vi "DataViewer_Transport.vi"() -> ()   [LabVIEW 2019]
uses:
  <userlib>/LevyLab/XY Utilities/subVIs/Waveform to XY (multiple).vi
  <userlib>/LevyLab/XY Utilities/subVIs/Waveform to XY (single).vi
  <vilib>/Waveform/WDTOps.llb/Waveform to XY Pairs.vi
  <vilib>/Waveform/WDTOps.llb/WDT Waveform to XY Pairs DBL.vi
  <userlib>/LevyLab/XY Utilities/xy_utilities.lvlib
panel:
  in  "Excitation (V)":dbl format="%#_6p"
  in  "Plot XG":bool
  in  "Plot XR":bool
  in  "V-":u16(ring) items=["", "Time", "Temperature", "AO1", "AO2", "AO3", "AO4", "AO5", "AO6", "AO7", "AO8", "AO9", "AO10", "AI1", "AI2", "AI3", "AI4", "AI5", "AI6", "AI7", "AI8", "AI9", "AI10", "X1", "X2", "X3", "X4", "X5", "X6", "X7", "X8", "X9", "X10", "Y1", "Y2", "Y3", "Y4", "Y5", "Y6", "Y7", "Y8", "Y9", "Y10"]
  in  "V+":u16(ring) items=["", "Time", "Temperature", "AO1", "AO2", "AO3", "AO4", "AO5", "AO6", "AO7", "AO8", "AO9", "AO10", "AI1", "AI2", "AI3", "AI4", "AI5", "AI6", "AI7", "AI8", "AI9", "AI10", "X1", "X2", "X3", "X4", "X5", "X6", "X7", "X8", "X9", "X10", "Y1", "Y2", "Y3", "Y4", "Y5", "Y6", "Y7", "Y8", "Y9", "Y10"]
  out "XY Graph":cluster{"Y-array":dbl[], "Y-array":dbl[]}(graph) caption="XY Graph - Light"
  in  "Y (or I- for XR/XG)":u16(ring) items=["", "Time", "Temperature", "AO1", "AO2", "AO3", "AO4", "AO5", "AO6", "AO7", "AO8", "AO9", "AO10", "AI1", "AI2", "AI3", "AI4", "AI5", "AI6", "AI7", "AI8", "AI9", "AI10", "X1", "X2", "X3", "X4", "X5", "X6", "X7", "X8", "X9", "X10", "Y1", "Y2", "Y3", "Y4", "Y5", "Y6", "Y7", "Y8", "Y9", "Y10"]
  in  "X":u16(ring) items=["", "Time", "Temperature", "AO1", "AO2", "AO3", "AO4", "AO5", "AO6", "AO7", "AO8", "AO9", "AO10", "AI1", "AI2", "AI3", "AI4", "AI5", "AI6", "AI7", "AI8", "AI9", "AI10", "X1", "X2", "X3", "X4", "X5", "X6", "X7", "X8", "X9", "X10", "Y1", "Y2", "Y3", "Y4", "Y5", "Y6", "Y7", "Y8", "Y9", "Y10"]
  in  "Plot XY":bool
  out "Experiment Notes":string
  in  "Open FIle":bool
  in  "File Path":path
  in  "Exit":bool
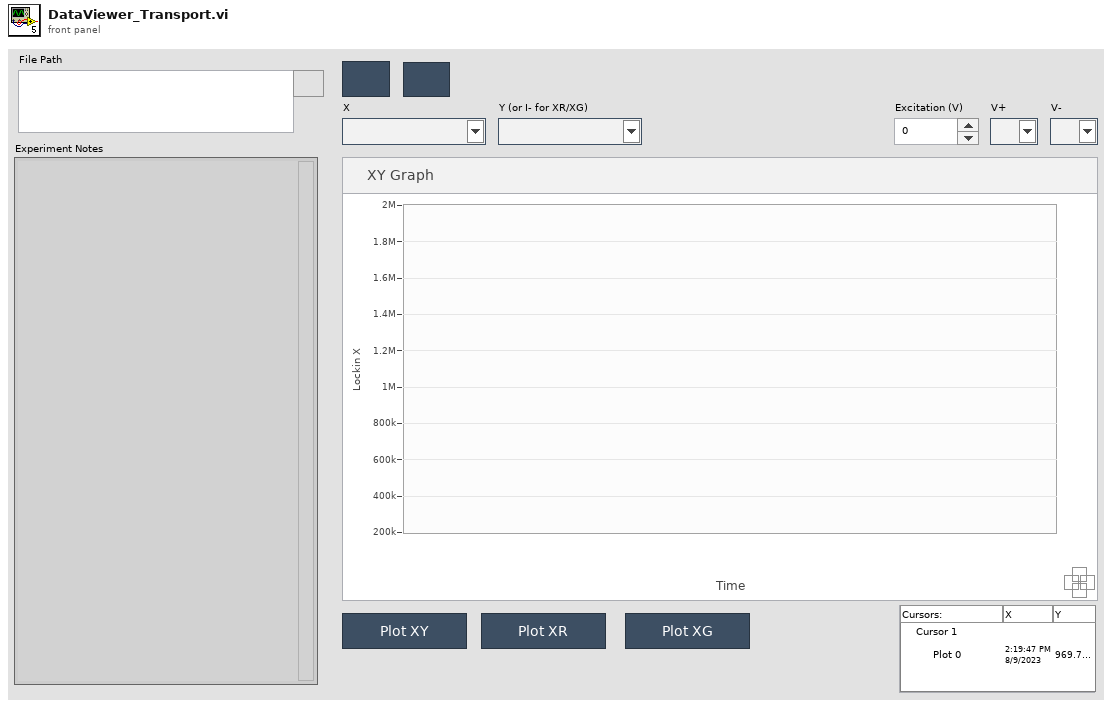
[diagram p1: front panel]
types:
  T1 = enum32{"Invalid", "Standard", "Closed", "Hidden", "Minimized", "Maximized"}
  T2 = enum32{"invalid app kind", "Development System", "Run Time System", "Student Edition", "Embedded LabVIEW", "Evaluation", "Custom"}
  T3 = cluster{"Core":cluster{"Current VI Reference":refnum<vi>, "Close Panel on Exit?":bool}, "Your Boolean data":bool, "Your string data":string, "TDMS Ref":refnum<k34>}
  T4 = cluster{"Current VI Reference":refnum<vi>, "Close Panel on Exit?":bool}
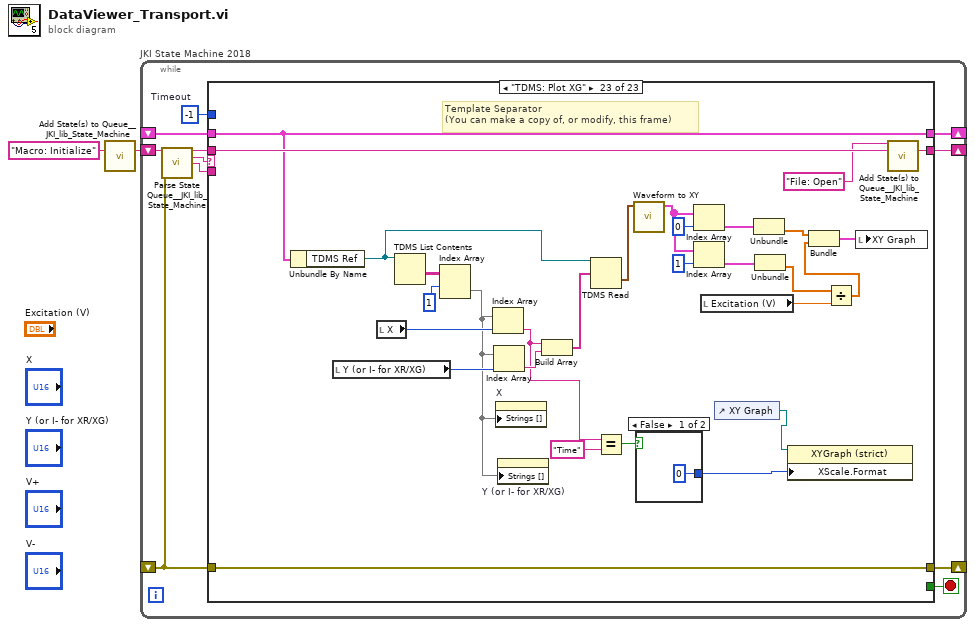
[diagram p0: block diagram]
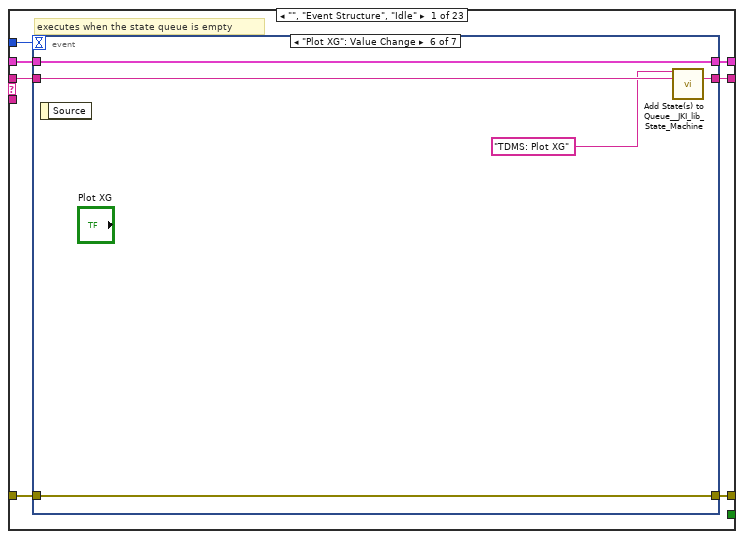
[diagram p2: hidden frame]
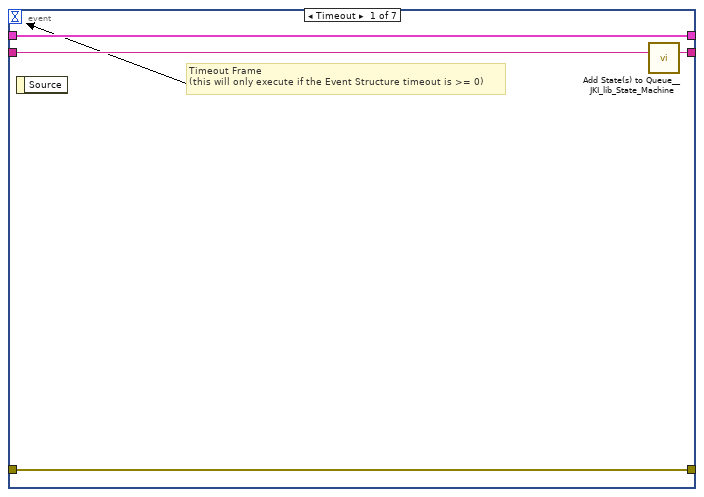
[diagram p3: hidden frame]
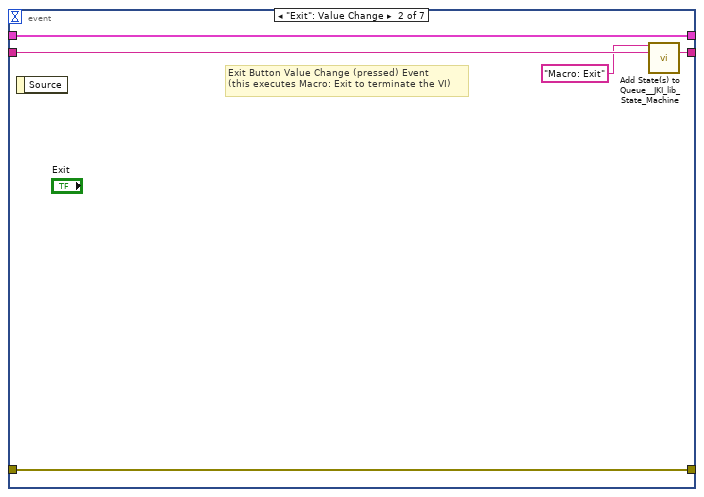
[diagram p4: hidden frame]
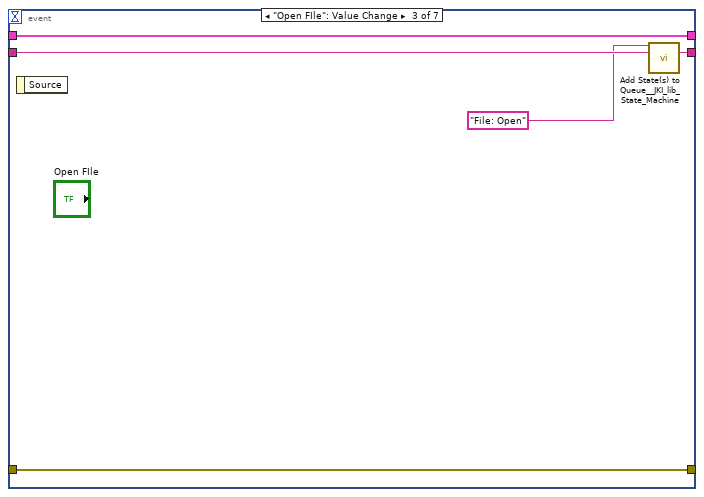
[diagram p5: hidden frame]
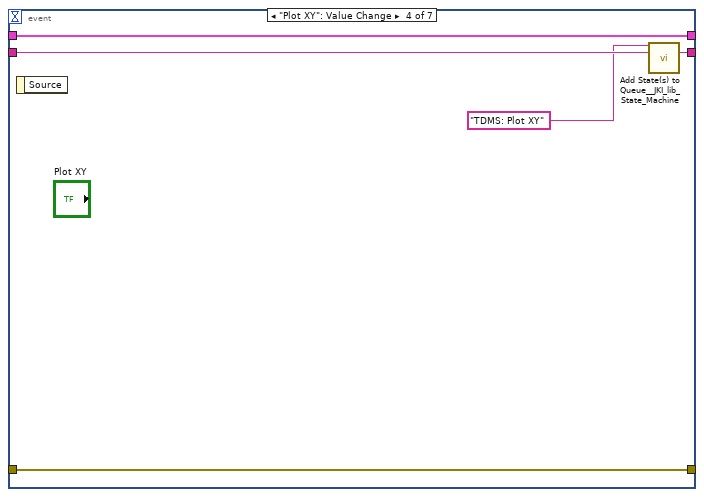
[diagram p6: hidden frame]
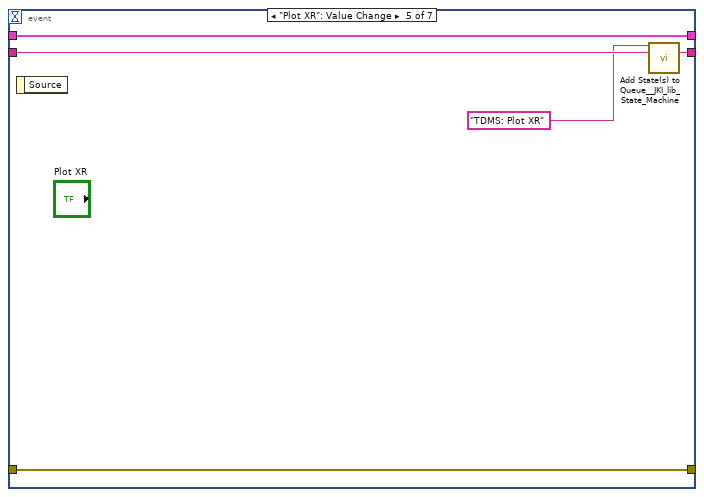
[diagram p7: hidden frame]
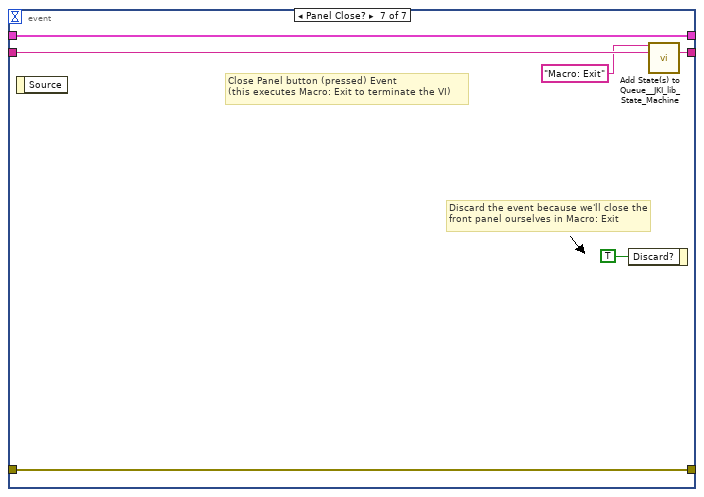
[diagram p8: hidden frame]
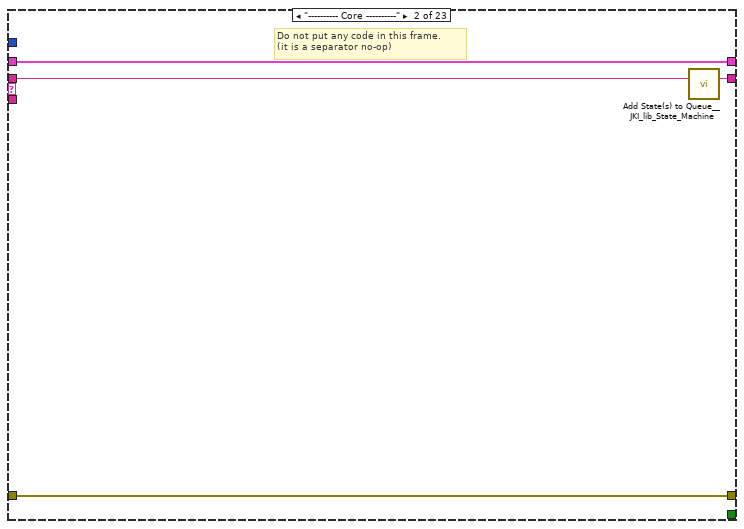
[diagram p9: hidden frame]
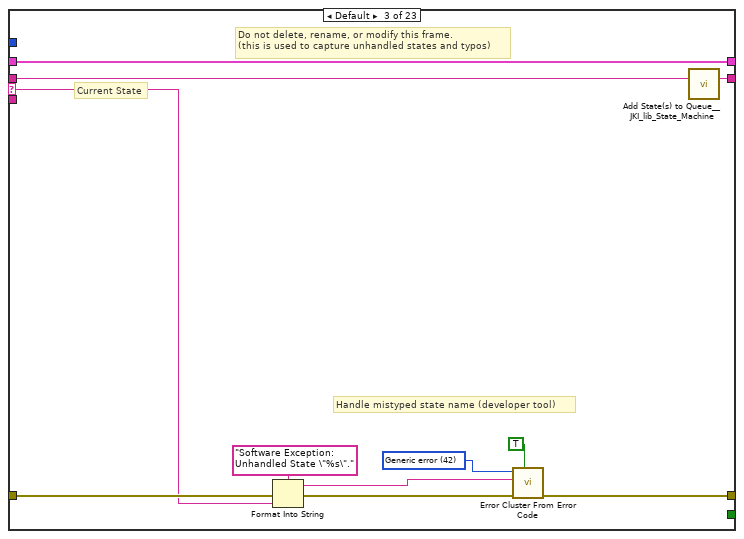
[diagram p10: hidden frame]
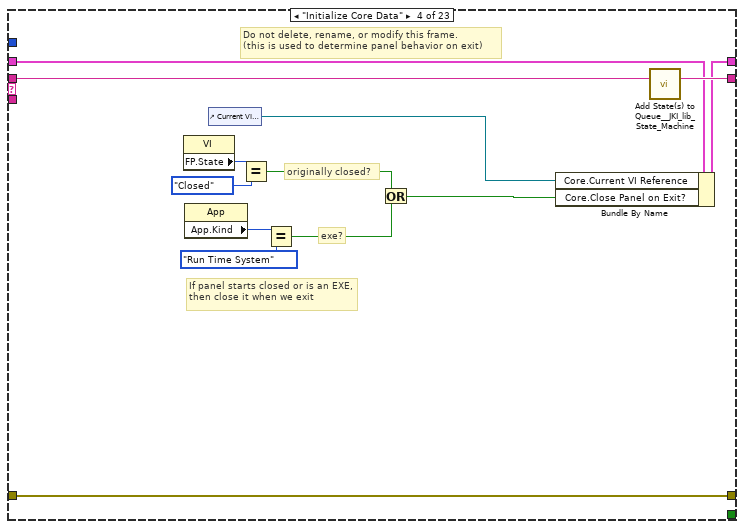
[diagram p11: hidden frame]
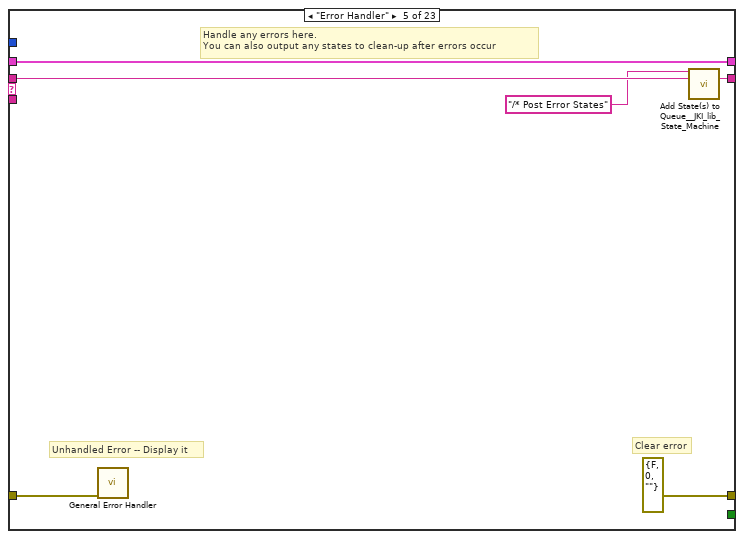
[diagram p12: hidden frame]
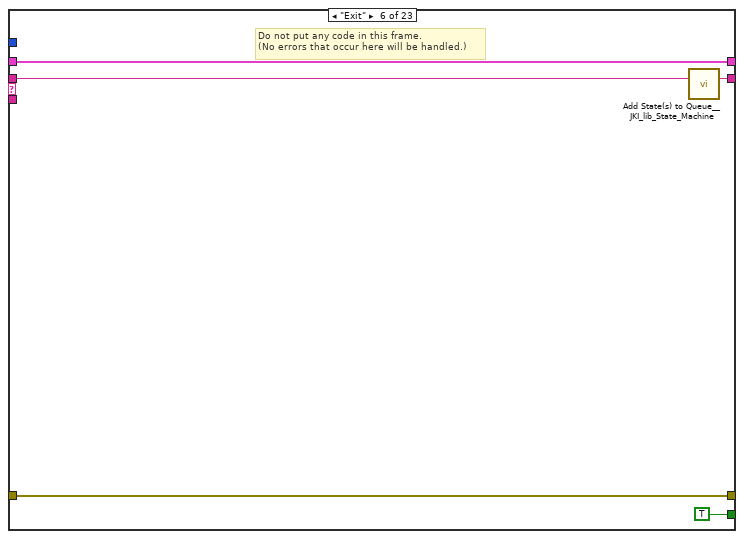
[diagram p13: hidden frame]
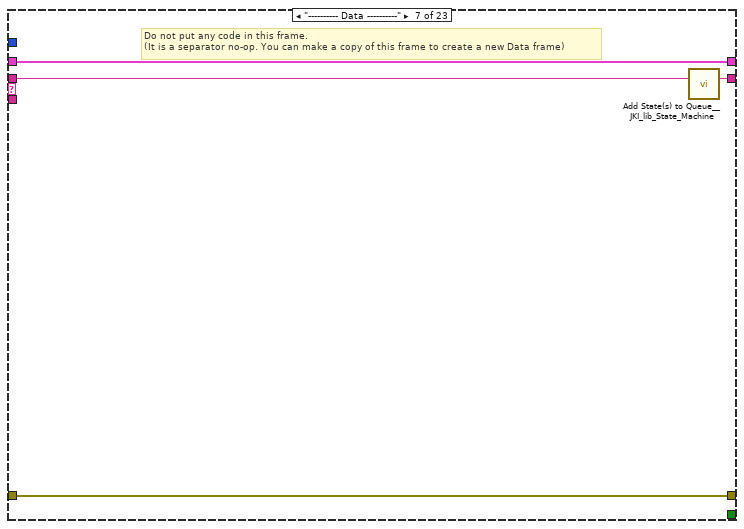
[diagram p14: hidden frame]
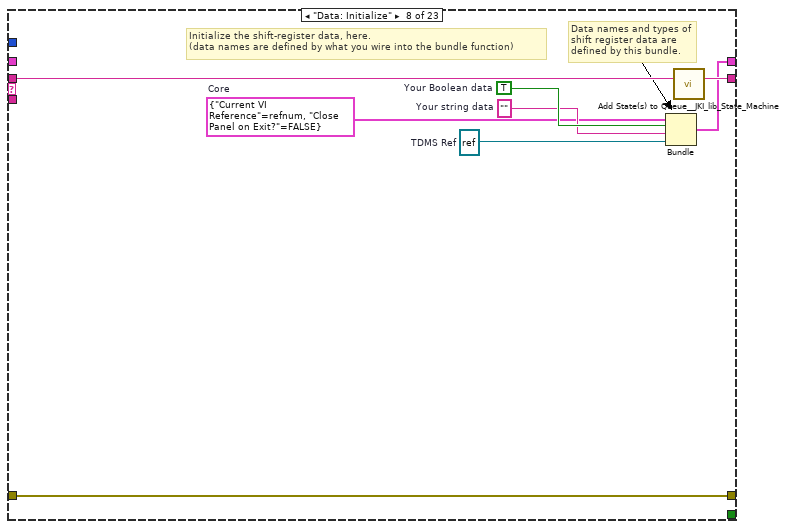
[diagram p15: hidden frame]
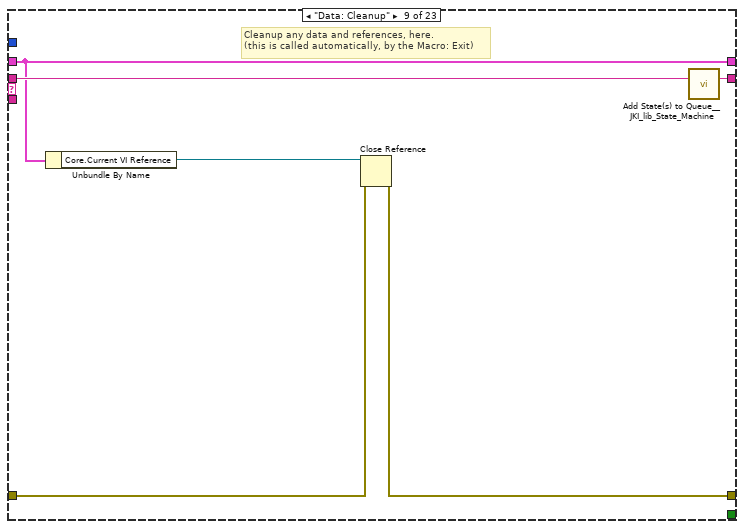
[diagram p16: hidden frame]
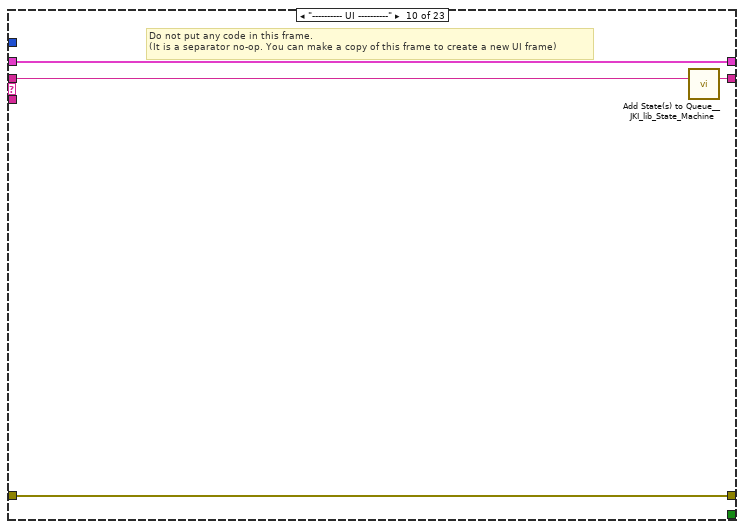
[diagram p17: hidden frame]
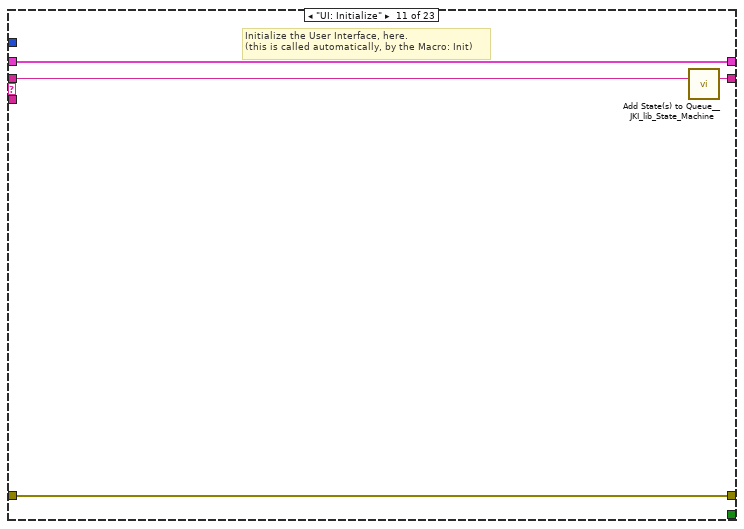
[diagram p18: hidden frame]
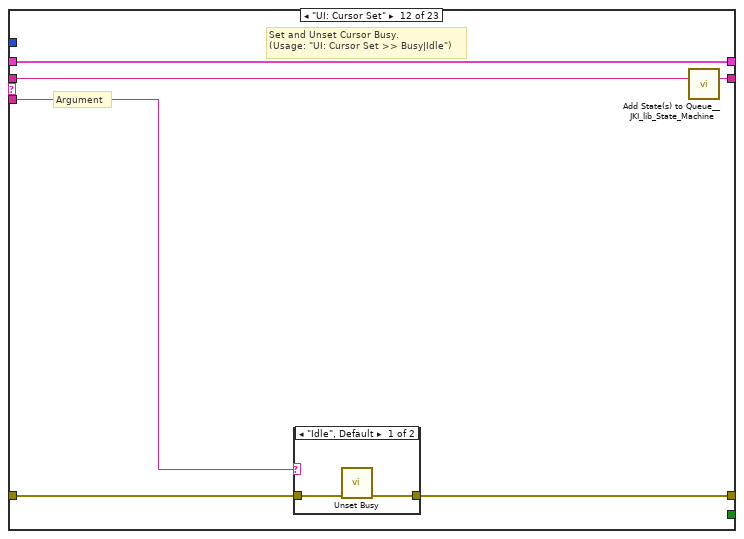
[diagram p19: hidden frame]
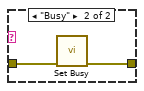
[diagram p20: hidden frame]
diagram:
  n1 = call <vilib>:"Add State(s) to Queue__JKI_lib_State_Machine.vi"("State(s) in (\"\")"="Macro: Initialize") -> ("States Out"=w2:string)  [unwired: 14 in]
  n2 = while "JKI State Machine 2018" {
    shift-right: [w6] -> _
    shift-left: _ -> [w5]
    shift-right: [w9] -> _
    shift-left: _ -> [w3]
    shift-right: [w8] -> _
    shift-left: w2 -> [w10]
    stop <- w7 stop-if-true
    w4 = -1  # Timeout
    n3 = call <vilib>:"Parse State Queue__JKI_lib_State_Machine.vi"("State Queue"=w10, "Error In (no error)"=w3) -> ("Remaining States"=w12:string, "Current State"=w13:string, "Arguments"=w11:string)  [unwired: 11 in]
    n4 = case shown="\"TDMS: Plot XG\"" w13 {
      selector: w13 -> [_ _ w60 _ _ _ _ _ _ _ _ _ _ _ _ _ _ _ _ _ _ _ _]
      tunnel: w12 -> [w20 w59 w64 w83 w89 w94 w98 w106 w112 w116 w120 w126 w137 w206 w211 w221 w225 w238 w246 w250 w276 w307 w338]
      tunnel: w11 -> [_ _ _ _ _ _ _ _ _ _ _ w121 w131 _ _ _ _ _ _ _ _ _ _]
      tunnel: w5 -> [w18 w56 w62 w76 w86 w92 w95 _ w107 w113 w118 w124 w133 w203 w208 w218 w222 w234 w242 w247 w273 w304 w335]
      tunnel: [w17 w57 w66 w80 errorcluster {"status"=FALSE, "code"=0, "source"=""} ("error out") w91 w96 w103 w108 w114 w117 w122 w134 w204 w209 w219 w223 w227 w239 w248 w274 w305 w336] -> w9
      tunnel: w3 -> [w16 w57 w65 w80 w85 w91 w96 w103 w109 w114 w117 w123 w135 w204 w209 w219 w223 w235 w240 w248 w274 w305 w336]
      tunnel: [w19 w58 w63 w82 w88 w93 w97 w105 w111 w115 w119 w125 w136 w205 w210 w220 w224 w237 w245 w249 w275 w306 w337] -> w8
      tunnel: [_ _ _ _ _ TRUE _ _ _ _ _ _ _ _ _ _ _ _ _ _ _ _ _] -> w7
      tunnel: [w15 w56 w62 w81 w86 w92 w95 w104 w107 w113 w118 w124 w133 w203 w208 w218 w222 w233 w244 w247 w273 w304 w335] -> w6
      tunnel: w4 -> [w14 _ _ _ _ _ _ _ _ _ _ _ _ _ _ _ _ _ _ _ _ _ _]
      frame "", "Event Structure", "Idle" {
        # "executes when the state queue is empty"
        n5 = event shown="[5] \"Plot XG\": Value Change" {
          selector: _ -> [_ _ _ _ _ _ _]
          dyn-events: _ -> [_ _ _ _ _ _ _]
          timeout: w14 -> [_ _ _ _ _ _ _]
          tunnel: w20 -> [w24 w29 w34 w39 w44 w49 w55]
          tunnel: [w23 w28 w33 w38 w43 w48 w54] -> w19
          tunnel: w18 -> [w21 w26 w31 w36 w41 w46 w52]
          tunnel: [w22 w27 w32 w37 w42 w47 w53] -> w17
          tunnel: w16 -> [w22 w27 w32 w37 w42 w47 w53]
          tunnel: [w21 w26 w31 w36 w41 w46 w52] -> w15
          event Timeout {
            # "Timeout Frame\n(this will only execute if the Event Structure timeout is >= 0)"
            n6 = event-data() -> ()  [unwired: 1 in, 1 out]
            n7 = call <vilib>:"Add State(s) to Queue__JKI_lib_State_Machine.vi"("State(s) in (\"\")"=w24) -> ("States Out"=w23:string)  [unwired: 14 in]
          }
          event "Exit": Value Change {
            # "Exit Button Value Change (pressed) Event\n(this executes Macro: Exit to terminate the VI)"
            n8 = event-data() -> ()  [unwired: 1 in, 1 out]
            n9 = call <vilib>:"Add State(s) to Queue__JKI_lib_State_Machine.vi"("State(s) in Front (\"\")"="Macro: Exit", "State(s) in (\"\")"=w29) -> ("States Out"=w28:string)  [unwired: 13 in]
          }
          event "Open FIle": Value Change {
            n10 = event-data() -> ()  [unwired: 1 in, 1 out]
            n11 = call <vilib>:"Add State(s) to Queue__JKI_lib_State_Machine.vi"("State(s) in Front (\"\")"="File: Open", "State(s) in (\"\")"=w34) -> ("States Out"=w33:string)  [unwired: 13 in]
          }
          event "Plot XY": Value Change {
            n12 = event-data() -> ()  [unwired: 1 in, 1 out]
            n13 = call <vilib>:"Add State(s) to Queue__JKI_lib_State_Machine.vi"("State(s) in Front (\"\")"="TDMS: Plot XY", "State(s) in (\"\")"=w39) -> ("States Out"=w38:string)  [unwired: 13 in]
          }
          event "Plot XR": Value Change {
            n14 = event-data() -> ()  [unwired: 1 in, 1 out]
            n15 = call <vilib>:"Add State(s) to Queue__JKI_lib_State_Machine.vi"("State(s) in Front (\"\")"="TDMS: Plot XR", "State(s) in (\"\")"=w44) -> ("States Out"=w43:string)  [unwired: 13 in]
          }
          event "Plot XG": Value Change {
            n16 = event-data() -> ()  [unwired: 1 in, 1 out]
            n17 = call <vilib>:"Add State(s) to Queue__JKI_lib_State_Machine.vi"("State(s) in Front (\"\")"="TDMS: Plot XG", "State(s) in (\"\")"=w49) -> ("States Out"=w48:string)  [unwired: 13 in]
          }
          event Panel Close? {
            # "Discard the event because we'll close the front panel ourselves in Macro: Exit"
            # "Close Panel button (pressed) Event\n(this executes Macro: Exit to terminate the VI)"
            n18 = event-data() -> ()  [unwired: 1 in, 1 out]
            n19 = event-data("Discard?"=TRUE) -> ()  [unwired: 1 in, 1 out]
            n20 = call <vilib>:"Add State(s) to Queue__JKI_lib_State_Machine.vi"("State(s) in Front (\"\")"="Macro: Exit", "State(s) in (\"\")"=w55) -> ("States Out"=w54:string)  [unwired: 13 in]
          }
        }
      }
      frame "---------- Core ----------" {
        # "Do not put any code in this frame.\n(it is a separator no-op)"
        n21 = call <vilib>:"Add State(s) to Queue__JKI_lib_State_Machine.vi"("State(s) in (\"\")"=w59) -> ("States Out"=w58:string)  [unwired: 14 in]
      }
      frame Default {
        w69 = 42 items=["No error", "Argument error", "Memory is full", "Out of zone", "End of file", "File already open", "Generic file I/O error", "File not found", "File permission error", "Disk is full", "Duplicate path", "Too many files open", "System feature not enabled", "Resource file not found", "Cannot add resource", "Resource not found", "Image not found", "Image memory error", "Pen does not exist", "Config type invalid", "Config token not found", "Config parse error", "Config memory error", "Bad external code format", "Bad external code offset", "External code not present", "Null window", "Destroy window error", "Null menu", "Print aborted", "Bad print record", "Print driver error", "Windows error during printing", "Memory error during printing", "Print dialog error", "Generic print error", "Invalid device refnum", "Device not found", "Device parameter error", "Device unit error", "Cannot open device", "Device call aborted", "Generic error", "Cancelled by user", "Object ID too low", "Object ID too high", "Object not in heap", "Unknown heap", "Unknown object (invalid DefProc)", "Unknown object (DefProc not in table)", "Message out of range", "Invalid (null) method", "Unknown message", "Manager call not supported", "Bad address", "Network operation in progress", "Network operation timed out", "Connection is busy", "Network attribute not supported", "Network error", "Address in use", "System out of memory", "Connection aborted", "Connection refused", "Not connected", "Already connected", "Connection closed", "Initialization error (interapplication manager)", "Bad occurrence", "Wait on unbound occurrence handler", "Occurrence queue overflow", "Datalog type conflict", "Unused", "Unrecognized type (interapplication manager)", "Memory corrupt", "Failed to make temporary DLL", "Old CIN version", "Drag socket not found", "Failed to load drop-object", "Failed to register OLE object", "Failed to release OLE object", "Format specifier type mismatch", "Unknown format specifier", "Too few format specifiers", "Too many format specifiers", "Scan failed", "Newer CIN version", "Error converting to variant", "Runtime menu error", "Password tampered", "Variant attribute not found", "Incompatible variant data type", "Event data is not available", "Event Store is not present", "Occurrence is not found", "Event Queue is not created", "Event info is not available", "Refnum passed is NULL", "Error retrieving Class GUID", "Error retrieving CoClass GUID", "Error retrieving TypeLib GUID.", "Bad built application magic bytes.", "Specific driver is different from the specific driver associated with the Logical Name.", "There is no session opened to the class driver.", "Max Error", "MAX - Error with config objects", "MAX - Error loading configuration", "MAX - Group not supported"]
        # "Current State"
        # "Do not delete, rename, or modify this frame.\n(this is used to capture unhandled states and typos)"
        # "Handle mistyped state name (developer tool)"
        n22 = Format Into String(format string="Software Exception: Unhandled State \"%s\"." ("message"), error in=w65, w60) -> (resulting string=w68:string, error out=w67:errorcluster)  [unwired: 1 in]
        n23 = call <vilib>:"Error Cluster From Error Code.vi"("show call chain? (False)"=TRUE, "error in (no error)"=w67, "error message (\"\")"=w68, "error code (0)"=w69) -> ("error out"=w66:errorcluster)  [unwired: 5 in]
        n24 = call <vilib>:"Add State(s) to Queue__JKI_lib_State_Machine.vi"("State(s) in (\"\")"=w64) -> ("States Out"=w63:string)  [unwired: 14 in]
      }
      frame "Initialize Core Data" {
        # "Do not delete, rename, or modify this frame.\n(this is used to determine panel behavior on exit)"
        # "originally closed?"
        # "exe?"
        # "If panel starts closed or is an EXE, then close it when we exit"
        n25 = property class="VI"() -> ("FP.State"=w73:T1)  [unwired: 2 in, 2 out]
        n26 = property class="App"() -> ("App.Kind"=w79:T2)  [unwired: 2 in, 2 out]
        n27 = control-ref of="Current VI Reference"() -> (w74:refnum<vi>)
        n28 = Equal?(x=w73, y=T1."Closed" ("Front Panel Window:State")) -> (x = y?=w71:bool)
        n29 = Equal?(x=w79, y=T2."Run Time System" ("Application:Kind")) -> (x = y?=w77:bool)
        n30 = Or(x=w71, y=w77) -> (x .or. y?=w75:bool)
        n31 = Bundle By Name(cluster=w76, "Core.Current VI Reference"=w74, "Core.Close Panel on Exit?"=w75) -> (w81:T3)
        n32 = call <vilib>:"Add State(s) to Queue__JKI_lib_State_Machine.vi"("State(s) in (\"\")"=w83) -> ("States Out"=w82:string)  [unwired: 14 in]
      }
      frame "Error Handler" {
        # "Unhandled Error -- Display it"
        # "Handle any errors here.\nYou can also output any states to clean-up after errors occur"
        # "Clear error"
        n33 = call <vilib>:"General Error Handler.vi"("error in (no error)"=w85) -> ()  [unwired: 10 in, 5 out]
        n34 = call <vilib>:"Add State(s) to Queue__JKI_lib_State_Machine.vi"("State(s) in Front (\"\")"="/* Post Error States", "State(s) in (\"\")"=w89) -> ("States Out"=w88:string)  [unwired: 13 in]
      }
      frame "Exit" {
        # "Do not put any code in this frame.\n(No errors that occur here will be handled.)"
        n35 = call <vilib>:"Add State(s) to Queue__JKI_lib_State_Machine.vi"("State(s) in (\"\")"=w94) -> ("States Out"=w93:string)  [unwired: 14 in]
      }
      frame "---------- Data ----------" {
        # "Do not put any code in this frame.\n(It is a separator no-op. You can make a copy of this frame to create a new Data frame)"
        n36 = call <vilib>:"Add State(s) to Queue__JKI_lib_State_Machine.vi"("State(s) in (\"\")"=w98) -> ("States Out"=w97:string)  [unwired: 14 in]
      }
      frame "Data: Initialize" {
        w99 = refnum<k34> refnum  # TDMS Ref
        w100 = T4 {"Current VI Reference"=refnum, "Close Panel on Exit?"=FALSE}  # Core
        w102 = TRUE  # Your Boolean data
        w101 = ""  # Your string data
        # "Data names and types of shift register data are defined by this bundle."
        # "Initialize the shift-register data, here.\n(data names are defined by what you wire into the bundle function)"
        n37 = Bundle("Core"=w100, "Your Boolean data"=w102, "Your string data"=w101, "TDMS Ref"=w99) -> (w104:T3)  [unwired: 1 in]
        n38 = call <vilib>:"Add State(s) to Queue__JKI_lib_State_Machine.vi"("State(s) in (\"\")"=w106) -> ("States Out"=w105:string)  [unwired: 14 in]
      }
      frame "Data: Cleanup" {
        # "Cleanup any data and references, here.\n(this is called automatically, by the Macro: Exit)"
        n39 = Unbundle By Name(w107) -> ("Core.Current VI Reference"=w110:refnum<vi>)
        n40 = Close Reference(reference=w110, error in (no error)=w109) -> (error out=w108:errorcluster)
        n41 = call <vilib>:"Add State(s) to Queue__JKI_lib_State_Machine.vi"("State(s) in (\"\")"=w112) -> ("States Out"=w111:string)  [unwired: 14 in]
      }
      frame "---------- UI ----------" {
        # "Do not put any code in this frame.\n(It is a separator no-op. You can make a copy of this frame to create a new UI frame)"
        n42 = call <vilib>:"Add State(s) to Queue__JKI_lib_State_Machine.vi"("State(s) in (\"\")"=w116) -> ("States Out"=w115:string)  [unwired: 14 in]
      }
      frame "UI: Initialize" {
        # "Initialize the User Interface, here.\n(this is called automatically, by the Macro: Init)"
        n43 = call <vilib>:"Add State(s) to Queue__JKI_lib_State_Machine.vi"("State(s) in (\"\")"=w120) -> ("States Out"=w119:string)  [unwired: 14 in]
      }
      frame "UI: Cursor Set" {
        # "Argument"
        # "Set and Unset Cursor Busy.\n(Usage: \"UI: Cursor Set >> Busy|Idle\")"
        n44 = case shown="\"Idle\", Default" w121 {
          tunnel: w123 -> [w128 w130]
          tunnel: [w127 w129] -> w122
          frame "Idle", Default {
            n45 = call <vilib>:"Unset Busy.vi"("error in (no error)"=w128) -> ("error out"=w127:errorcluster)  [unwired: 10 in]
          }
          frame "Busy" {
            n46 = call <vilib>:"Set Busy.vi"("error in (no error)"=w130) -> ("error out"=w129:errorcluster)  [unwired: 9 in, 1 out]
          }
        }
        n47 = call <vilib>:"Add State(s) to Queue__JKI_lib_State_Machine.vi"("State(s) in (\"\")"=w126) -> ("States Out"=w125:string)  [unwired: 14 in]
      }
      frame "UI: Front Panel State" {
        # "Argument"
        # "Set Front Panel Open or Closed\n(Usage: \"UI: Front Panel State >> Open|Close\")"
        n48 = Unbundle By Name(w133) -> ("Core.Current VI Reference"=w132:refnum<vi>)
        n49 = case shown="\"Minimize\", \"Minimized\"" w131 {
          tunnel: w135 -> [w143 w158 w169 w182 w195]
          tunnel: [w145 w159 w171 w184 w197] -> w134
          tunnel: w132 -> [w144 w156 w170 w183 w196]
          frame "Open", "Standard", Default {
            w138 = T1."Standard" ("State")
            n50 = property class="VI"(reference=w144, error in=w143) -> (reference out=w141:refnum<vi>, error out=w142:errorcluster, "FP.State"=w140:T1)
            n51 = Not Equal?(x=w140, y=w138) -> (x != y?=w139:bool)
            n52 = case shown="True" w139 {
              tunnel: [w149 w151] -> w145
              tunnel: w142 -> [w148 w151]
              tunnel: w141 -> [w147 _]
              tunnel: w138 -> [w146 _]
              frame True {
                n53 = invoke class="VI" method="FP.Open"(reference=w147, error in=w148, "Activate"=TRUE, "State"=w146) -> (error out=w149:errorcluster)  [unwired: 1 in, 4 out]
              }
              frame False {
              }
            }
          }
          frame "Close", "Closed" {
            n54 = property class="VI"(reference=w156, error in=w158) -> (reference out=w155:refnum<vi>, error out=w157:errorcluster, "FP.State"=w153:T1)
            n55 = Not Equal?(x=w153, y=T1."Closed" ("Front Panel Window:State")) -> (x != y?=w152:bool)
            n56 = case shown="True" w152 {
              tunnel: [w160 w163] -> w159
              tunnel: w157 -> [w160 w162]
              tunnel: w155 -> [_ w161]
              frame False {
              }
              frame True {
                n57 = invoke class="VI" method="FP.Close"(reference=w161, error in=w162) -> (error out=w163:errorcluster)  [unwired: 1 in, 2 out]
              }
            }
          }
          frame "Hidden", "Hide" {
            w164 = T1."Hidden" ("State")
            n58 = property class="VI"(reference=w170, error in=w169) -> (reference out=w167:refnum<vi>, error out=w168:errorcluster, "FP.State"=w166:T1)
            n59 = Not Equal?(x=w166, y=w164) -> (x != y?=w165:bool)
            n60 = case shown="True" w165 {
              tunnel: [w175 w176] -> w171
              tunnel: w168 -> [w174 w176]
              tunnel: w167 -> [w173 _]
              tunnel: w164 -> [w172 _]
              frame True {
                n61 = invoke class="VI" method="FP.Open"(reference=w173, error in=w174, "State"=w172) -> (error out=w175:errorcluster)  [unwired: 2 in, 4 out]
              }
              frame False {
              }
            }
          }
          frame "Minimize", "Minimized" {
            w177 = T1."Minimized" ("State")
            n62 = property class="VI"(reference=w183, error in=w182) -> (reference out=w180:refnum<vi>, error out=w181:errorcluster, "FP.State"=w179:T1)
            n63 = Not Equal?(x=w179, y=w177) -> (x != y?=w178:bool)
            n64 = case shown="True" w178 {
              tunnel: [w188 w189] -> w184
              tunnel: w181 -> [w187 w189]
              tunnel: w180 -> [w186 _]
              tunnel: w177 -> [w185 _]
              frame True {
                n65 = invoke class="VI" method="FP.Open"(reference=w186, error in=w187, "State"=w185) -> (error out=w188:errorcluster)  [unwired: 2 in, 4 out]
              }
              frame False {
              }
            }
          }
          frame "Maximize", "Maximized" {
            w190 = T1."Maximized" ("State")
            n66 = property class="VI"(reference=w196, error in=w195) -> (reference out=w193:refnum<vi>, error out=w194:errorcluster, "FP.State"=w192:T1)
            n67 = Not Equal?(x=w192, y=w190) -> (x != y?=w191:bool)
            n68 = case shown="True" w191 {
              tunnel: [w201 w202] -> w197
              tunnel: w194 -> [w200 w202]
              tunnel: w193 -> [w199 _]
              tunnel: w190 -> [w198 _]
              frame True {
                n69 = invoke class="VI" method="FP.Open"(reference=w199, error in=w200, "State"=w198) -> (error out=w201:errorcluster)  [unwired: 2 in, 4 out]
              }
              frame False {
              }
            }
          }
        }
        n70 = call <vilib>:"Add State(s) to Queue__JKI_lib_State_Machine.vi"("State(s) in (\"\")"=w137) -> ("States Out"=w136:string)  [unwired: 14 in]
      }
      frame "---------- Macro ----------" {
        # "Do not put any code in this frame.\n(It is a separator no-op. You can make a copy of this frame to create a new Macro frame)"
        n71 = call <vilib>:"Add State(s) to Queue__JKI_lib_State_Machine.vi"("State(s) in (\"\")"=w206) -> ("States Out"=w205:string)  [unwired: 14 in]
      }
      frame "Macro: Initialize" {
        w207 = "Data: Initialize\nFile: Open\nInitialize Core Data\nUI: Initialize\nUI: Front Panel State >> Open"  # Data: Initialize File: Open Initialize Core Data UI: Initialize UI: Front Panel State >> Open
        # "Initialization Macro\n(This is called once, when the VI starts)"
        n72 = call <vilib>:"Add State(s) to Queue__JKI_lib_State_Machine.vi"("State(s) in Front (\"\")"=w207, "State(s) in (\"\")"=w211) -> ("States Out"=w210:string)  [unwired: 13 in]
      }
      frame "Macro: Exit" {
        # "Exit Macro\n(This is called once, when the VI exits)"
        n73 = Unbundle By Name(w218) -> ("Core.Close Panel on Exit?"=w217:bool)
        n74 = Select(t="UI: Front Panel State >> Close", s=w217, f="") -> (s? t:f=w214:string)
        n75 = call <vilib>:"Add State(s) to Queue__JKI_lib_State_Machine.vi"("State(s) in (\"\")"=w214, "State(s) at Back (\"\")"="Data: Cleanup\nFile: Close\nExit") -> ("States Out"=w212:string)  [unwired: 13 in]
        n76 = call <vilib>:"Add State(s) to Queue__JKI_lib_State_Machine.vi"("State(s) in Front (\"\")"=w212, "State(s) in (\"\")"=w221) -> ("States Out"=w220:string)  [unwired: 13 in]
      }
      frame "---------- File ----------" {
        # "Template Separator\n(You can make a copy of, or modify, this frame)"
        n77 = call <vilib>:"Add State(s) to Queue__JKI_lib_State_Machine.vi"("State(s) in (\"\")"=w225) -> ("States Out"=w224:string)  [unwired: 14 in]
      }
      frame "File: Open" {
        # "Your code here.\n(You can make a copy of, or modify, this frame)"
        n78 = TDMS Open(8:w235, 11:"File Path") -> (0:w228:errorcluster, 3:w226:refnum<k34>)  [unwired: 5 in]
        n79 = TDMS Get Properties(5:"" ("data type"), 7:"Notes" ("property name"), 8:w228, 11:w226) -> (0:w227:errorcluster, 4:→"Experiment Notes":string)  [unwired: 2 in, 4 out]
        n80 = Bundle By Name(cluster=w234, "TDMS Ref"=w226) -> (w233:T3)
        n81 = property on="Experiment Notes" class="Str"("VScrollVis"=TRUE ("Vertical Scrollbar Visible")) -> ()  [unwired: 2 in, 2 out]
        n82 = call <vilib>:"Add State(s) to Queue__JKI_lib_State_Machine.vi"("State(s) in (\"\")"=w238) -> ("States Out"=w237:string)  [unwired: 14 in]
      }
      frame "File: Close" {
        # "Your code here.\n(You can make a copy of, or modify, this frame)"
        n83 = Unbundle By Name(w242) -> ("TDMS Ref"=w241:refnum<k34>)
        n84 = TDMS Close(8:w240, 11:w241) -> (0:w239:errorcluster)  [unwired: 1 out]
        n85 = Bundle By Name(cluster=w242, "TDMS Ref"=refnum<k34> refnum) -> (w244:T3)
        n86 = call <vilib>:"Add State(s) to Queue__JKI_lib_State_Machine.vi"("State(s) in (\"\")"=w246) -> ("States Out"=w245:string)  [unwired: 14 in]
      }
      frame "---------- TDMS ----------" {
        # "Template Separator\n(You can make a copy of, or modify, this frame)"
        n87 = call <vilib>:"Add State(s) to Queue__JKI_lib_State_Machine.vi"("State(s) in (\"\")"=w250) -> ("States Out"=w249:string)  [unwired: 14 in]
      }
      frame "TDMS: Plot XY" {
        # "Template Separator\n(You can make a copy of, or modify, this frame)"
        n88 = Unbundle By Name(w273) -> ("TDMS Ref"=w271:refnum<k34>)
        n89 = local read "Y (or I- for XR/XG)"() -> (w265:u16)
        n90 = local read "X"() -> (w266:u16)
        n91 = TDMS List Contents(7:w271) -> (1:w272:string[][])  [unwired: 2 in, 3 out]
        n92 = Index Array(array=w272, index (row)=1) -> (element=w264:string[])  [unwired: 1 in]
        n93 = Index Array(array=w264, index=w266) -> (element=w253:string)
        n94 = Index Array(array=w264, index=w265) -> (element=w268:string)
        n95 = property on="X" class="Ring (strict)"("Strings []"=w264) -> ()  [unwired: 2 in, 2 out]
        n96 = property on="Y (or I- for XR/XG)" class="Ring (strict)"("Strings []"=w264) -> ()  [unwired: 2 in, 2 out]
        n97 = Build Array(w253, w268) -> (w267:string[])
        n98 = TDMS Read(0:w271, 7:w267) -> (10:w263:waveform(dbl)[])  [unwired: 6 in, 5 out]
        n99 = Equal?(x=w253, y="Time") -> (x = y?=w254:bool)
        n100 = case shown="False" w254 {
          tunnel: [u8 0 ("X Scale.Display Format:Format") u8 7 ("X Scale.Display Format:Format")] -> w251
          frame False {
          }
          frame True {
          }
        }
        n101 = call-poly <userlib>:"Waveform to XY.vi"("Waveform in"=w263) -> ("XY-data out"=w261:cluster{"X-array":dbl[], "Y-array":dbl[]}[])  [unwired: 9 in, 1 out]
        n102 = Index Array(array=w261, index=0) -> (element=w262:cluster{"X-array":dbl[], "Y-array":dbl[]})
        n103 = Index Array(array=w261, index=1) -> (element=w258:cluster{"X-array":dbl[], "Y-array":dbl[]})
        n104 = property on="XY Graph" class="XYGraph (strict)"("XScale.Format"=w251) -> ()  [unwired: 2 in, 2 out]
        n105 = Unbundle(w262) -> ("Y-array"=w257:dbl[])  [unwired: 1 out]
        n106 = Unbundle(w258) -> ("Y-array"=w256:dbl[])  [unwired: 1 out]
        n107 = Bundle("Y-array"=w257, "Y-array"=w256) -> (→"XY Graph":cluster{"Y-array":dbl[], "Y-array":dbl[]})  [unwired: 1 in]
        n108 = call <vilib>:"Add State(s) to Queue__JKI_lib_State_Machine.vi"("State(s) in Front (\"\")"="File: Open" ("State(s) in Front (\"\")"), "State(s) in (\"\")"=w276) -> ("States Out"=w275:string)  [unwired: 13 in]
      }
      frame "TDMS: Plot XR" {
        # "Template Separator\n(You can make a copy of, or modify, this frame)"
        n109 = Unbundle By Name(w304) -> ("TDMS Ref"=w302:refnum<k34>)
        n110 = local read "Y (or I- for XR/XG)"() -> (w296:u16)
        n111 = local read "X"() -> (w297:u16)
        n112 = TDMS List Contents(7:w302) -> (1:w303:string[][])  [unwired: 2 in, 3 out]
        n113 = Index Array(array=w303, index (row)=1) -> (element=w295:string[])  [unwired: 1 in]
        n114 = Index Array(array=w295, index=w297) -> (element=w286:string)
        n115 = Index Array(array=w295, index=w296) -> (element=w299:string)
        n116 = property on="X" class="Ring (strict)"("Strings []"=w295) -> ()  [unwired: 2 in, 2 out]
        n117 = property on="Y (or I- for XR/XG)" class="Ring (strict)"("Strings []"=w295) -> ()  [unwired: 2 in, 2 out]
        n118 = Build Array(w286, w299) -> (w298:string[])
        n119 = TDMS Read(0:w302, 7:w298) -> (10:w294:waveform(dbl)[])  [unwired: 6 in, 5 out]
        n120 = Equal?(x=w286, y="Time") -> (x = y?=w287:bool)
        n121 = call-poly <userlib>:"Waveform to XY.vi"("Waveform in"=w294) -> ("XY-data out"=w292:cluster{"X-array":dbl[], "Y-array":dbl[]}[])  [unwired: 9 in, 1 out]
        n122 = case shown="False" w287 {
          tunnel: [u8 0 ("X Scale.Display Format:Format") u8 7 ("X Scale.Display Format:Format")] -> w283
          frame False {
          }
          frame True {
          }
        }
        n123 = local read "Excitation (V)"() -> (w279:dbl)
        n124 = Index Array(array=w292, index=0) -> (element=w293:cluster{"X-array":dbl[], "Y-array":dbl[]})
        n125 = Index Array(array=w292, index=1) -> (element=w289:cluster{"X-array":dbl[], "Y-array":dbl[]})
        n126 = control-ref of="XY Graph"() -> (w282:refnum<vi>)
        n127 = Unbundle(w293) -> ("Y-array"=w288:dbl[])  [unwired: 1 out]
        n128 = Unbundle(w289) -> ("Y-array"=w281:dbl[])  [unwired: 1 out]
        n129 = property on="Property Node" class="XYGraph (strict)"(reference=w282, "XScale.Format"=w283) -> ()  [unwired: 1 in, 2 out]
        n130 = Divide(x=w279, y=w281) -> (x/y=w280:dbl[])
        n131 = Bundle("Y-array"=w288, w280) -> (w284:cluster{"Y-array":dbl[], dbl[]})  [unwired: 1 in]
        n132 = local write "XY Graph"(w284) -> ()
        n133 = call <vilib>:"Add State(s) to Queue__JKI_lib_State_Machine.vi"("State(s) in Front (\"\")"="File: Open" ("State(s) in Front (\"\")"), "State(s) in (\"\")"=w307) -> ("States Out"=w306:string)  [unwired: 13 in]
      }
      frame "TDMS: Plot XG" {
        # "Template Separator\n(You can make a copy of, or modify, this frame)"
        n134 = Unbundle By Name(w335) -> ("TDMS Ref"=w333:refnum<k34>)
        n135 = local read "Y (or I- for XR/XG)"() -> (w327:u16)
        n136 = local read "X"() -> (w328:u16)
        n137 = TDMS List Contents(7:w333) -> (1:w334:string[][])  [unwired: 2 in, 3 out]
        n138 = Index Array(array=w334, index (row)=1) -> (element=w326:string[])  [unwired: 1 in]
        n139 = Index Array(array=w326, index=w328) -> (element=w317:string)
        n140 = Index Array(array=w326, index=w327) -> (element=w330:string)
        n141 = property on="X" class="Ring (strict)"("Strings []"=w326) -> ()  [unwired: 2 in, 2 out]
        n142 = property on="Y (or I- for XR/XG)" class="Ring (strict)"("Strings []"=w326) -> ()  [unwired: 2 in, 2 out]
        n143 = Build Array(w317, w330) -> (w329:string[])
        n144 = TDMS Read(0:w333, 7:w329) -> (10:w325:waveform(dbl)[])  [unwired: 6 in, 5 out]
        n145 = Equal?(x=w317, y="Time") -> (x = y?=w318:bool)
        n146 = call-poly <userlib>:"Waveform to XY.vi"("Waveform in"=w325) -> ("XY-data out"=w323:cluster{"X-array":dbl[], "Y-array":dbl[]}[])  [unwired: 9 in, 1 out]
        n147 = case shown="False" w318 {
          tunnel: [u8 0 ("X Scale.Display Format:Format") u8 7 ("X Scale.Display Format:Format")] -> w315
          frame False {
          }
          frame True {
          }
        }
        n148 = Index Array(array=w323, index=0) -> (element=w324:cluster{"X-array":dbl[], "Y-array":dbl[]})
        n149 = Index Array(array=w323, index=1) -> (element=w320:cluster{"X-array":dbl[], "Y-array":dbl[]})
        n150 = local read "Excitation (V)"() -> (w311:dbl)
        n151 = control-ref of="XY Graph"() -> (w314:refnum<vi>)
        n152 = Unbundle(w324) -> ("Y-array"=w319:dbl[])  [unwired: 1 out]
        n153 = Unbundle(w320) -> ("Y-array"=w312:dbl[])  [unwired: 1 out]
        n154 = property on="Property Node" class="XYGraph (strict)"(reference=w314, "XScale.Format"=w315) -> ()  [unwired: 1 in, 2 out]
        n155 = Divide(x=w312, y=w311) -> (x/y=w313:dbl[])
        n156 = Bundle("Y-array"=w319, w313) -> (w310:cluster{"Y-array":dbl[], dbl[]})  [unwired: 1 in]
        n157 = local write "XY Graph"(w310) -> ()
        n158 = call <vilib>:"Add State(s) to Queue__JKI_lib_State_Machine.vi"("State(s) in Front (\"\")"="File: Open" ("State(s) in Front (\"\")"), "State(s) in (\"\")"=w338) -> ("States Out"=w337:string)  [unwired: 13 in]
      }
    }
  }
